vi "Create DVR.vi"(8 "error in (no error)":errorcluster, 11 "DispSnsr in":refnum<class "DispSnsr.lvclass">) -> (0 "error out":errorcluster, 2 "data value reference":refnum<data-value>, 3 "DispSnsr out":refnum<class "DispSnsr.lvclass">)   [LabVIEW 2016, in "Hardware.lvlib" / "Displacement Sensor.lvlib" / "DispSnsr.lvclass"]
uses:
  <userlib>/Common Components/Hardware/Displacement Sensor/DispSnsr/DispSnsr.lvclass
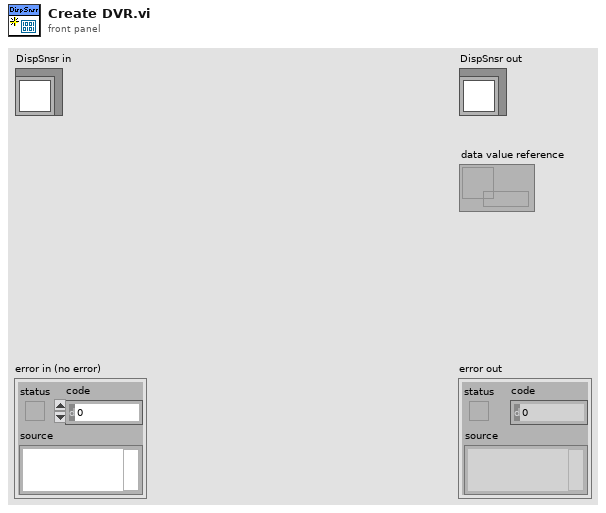
[diagram p1: front panel]
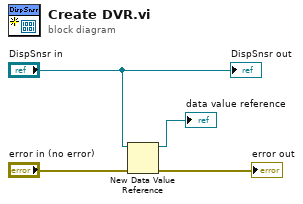
[diagram p0: block diagram]
diagram:
  n1 = New Data Value Reference(data value="DispSnsr in", error in="error in (no error)") -> (data value reference=→"data value reference":refnum<data-value>, error out=→"error out":errorcluster)
  "DispSnsr out" <- "DispSnsr in"
